vi "Locked Rotor.vi"(0 "GEA2 Reference In":refnum<k24>, 1 "Mode":T1, 2 "Hall Speed (RPM)":dbl=15.0, 3 "Previous Fault Count":u8, 5 "Standalone?":bool, 7 "GEA Inputs":T2={"Source"=228, "Destination"=32} {"Destination" format="%.0x"; "Source" format="%.0x"}, 11 "Error In":errorcluster, 12 "Counter":tag, 13 "Hall Sensor Channel":tag) -> (4 "GEA2 Reference Out":refnum<k24>, 6 "Pass/Fail?":bool, 8 "Report Text":string, 10 "Current Fault Count":u8, 15 "Error Out":errorcluster)   [LabVIEW 2016, in "TLMB.lvlib"]
doc: "This VI tests the locked rotor fault detection algorithm. It can be used to test in spin or agitate. QA XML must be used and test can only be executed on the soft load box (SLB)."
uses:
  Projects/TLMB.lvlib
  Q:/Common/DLLs/GEA3/GeaCommunication.dll
  Common/DLLs/GEA3/GeaCommunication.dll
  Common/LabVIEW GEA2 Toolkit/LabVIEW_GEA2_Toolkit.lvlibp/type defs/Source_Destination.ctl
  controls/Mode.ctl
  Common/LabVIEW GEA2 Toolkit/LabVIEW_GEA2_Toolkit.lvlibp/type defs/ERD Read Data In.ctl
  Common/LabVIEW GEA2 Toolkit/LabVIEW_GEA2_Toolkit.lvlibp/type defs/Data Type.ctl
  Common/LabVIEW GEA2 Toolkit/LabVIEW_GEA2_Toolkit.lvlibp/type defs/ERD Write Data In.ctl
  <vilib>/DAQmx/create/channels.llb/DAQmx Create Channel (CO-Pulse Generation-Frequency).vi
  <vilib>/DAQmx/configure/timing.llb/DAQmx Timing (Implicit).vi
  Common/LabVIEW GEA2 Toolkit/LabVIEW_GEA2_Toolkit.lvlibp
  <resource>/objmgr/daqmx.rc
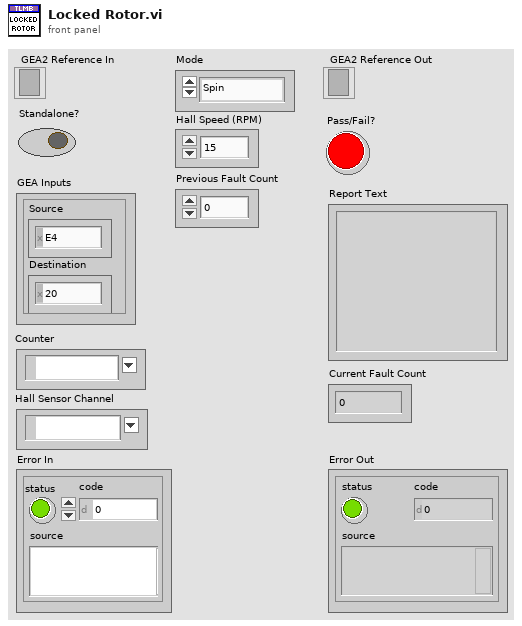
[diagram p1: front panel]
types:
  T1 = typedef "TLMB.lvlib/Mode.ctl" = enum16{"Spin", "Agitate"}
  T2 = typedef "LabVIEW_GEA2_Toolkit.lvlibp/Source_Destination.ctl" = cluster{"Source":u8, "Destination":u8}
  T3 = typedef "LabVIEW_GEA2_Toolkit.lvlibp/ERD Read Data In.ctl" = cluster{"ERD Number":u16, "Data Type":T4}
  T4 = typedef "LabVIEW_GEA2_Toolkit.lvlibp/Data Type.ctl" = enum16{"string", "boolean", "uint8_t", "uint16_t", "uint32_t", "uint64_t", "int8_t", "int16_t", "int32_t", "int64_t"}
  T5 = typedef "LabVIEW_GEA2_Toolkit.lvlibp/ERD Write Data In.ctl" = cluster{"ERD Number":u16, "Data Type":T4, "Data":string}
  T6 = typedef "LabVIEW_GEA2_Toolkit.lvlibp/ERD Read Data Out.ctl" = cluster{"ERD Number":u16, "Data":string}
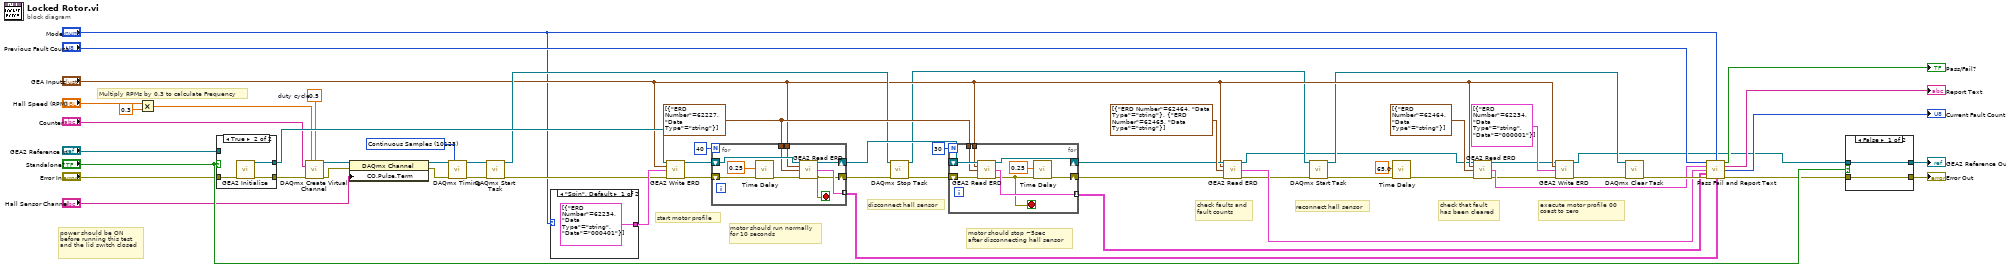
[diagram p0: block diagram]
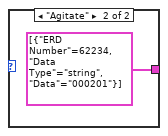
[diagram p2: hidden frame]
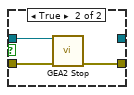
[diagram p3: hidden frame]
diagram:
  w42 = 0.5  # duty cycle
  w39 = T3[] [{"ERD Number"=62227, "Data Type"=enum."string"}] ("Read ERD List")
  w51 = 10123 items=["Finite Samples"=10178, "Continuous Samples"=10123, "Hardware Timed Single Point"=12522] ("sample mode")
  # "Multiply RPMs by 0.3 to calculate Frequency"
  # "check that fault\nhas been cleared"
  # "check faults and\nfault counts"
  # "reconnect hall sensor"
  # "power should be ON\nbefore running this test\nand the lid switch closed"
  # "execute motor profile 00\ncoast to zero"
  # "motor should stop ~5sec\nafter disconnecting hall sensor"
  # "start motor profile"
  # "motor should run normally\nfor 10 seconds"
  # "disconnect hall sensor"
  n1 = Multiply(x="Hall Speed (RPM)", y=0.3) -> (x*y=w43:dbl)
  n2 = case shown="True" "Standalone?" {
    tunnel: [w60 w64] -> w57
    tunnel: [w61 w63] -> w11
    tunnel: "Error In" -> [w61 w62]
    tunnel: "GEA2 Reference In" -> [w60 _]
    frame False {
    }
    frame True {
      n3 = call "GEA2 Initialize.vi"("error in"=w62) -> ("GEA2 Reference Out"=w64:refnum<k24>, "error out"=w63:errorcluster)  [unwired: 12 in, 1 out]
    }
  }
  n4 = call-poly <vilib>:"DAQmx Create Virtual Channel.vi"("frequency"=w43, "duty cycle"=w42, "counter"="Counter", "error in"=w11) -> ("task out"=w55:refnum<k21>, "error out"=w54:errorcluster)  [unwired: 10 in]
  n5 = property class="DAQmx Channel"(reference=w55, error in=w54, "CO.Pulse.Term"="Hall Sensor Channel") -> (reference out=w53:refnum<k21>, error out=w52:errorcluster)
  n6 = call-poly <vilib>:"DAQmx Timing.vi"("task/channels in"=w53, "sample mode"=w51, "error in"=w52) -> ("task out"=w50:refnum<k21>, "error out"=w49:errorcluster)  [unwired: 11 in]
  n7 = call <vilib>:"DAQmx Start Task.vi"("task/channels in"=w50, "error in"=w49) -> ("task out"=w33:refnum<k21>, "error out"=w48:errorcluster)  [unwired: 12 in]
  n8 = case shown="\"Spin\", Default" "Mode" {
    tunnel: [T5[] [{"ERD Number"=62234, "Data Type"=enum."string", "Data"="000401"}] ("Write ERD List") T5[] [{"ERD Number"=62234, "Data Type"=enum."string", "Data"="000201"}] ("Write ERD List")] -> w56
    frame "Spin", Default {
    }
    frame "Agitate" {
    }
  }
  n9 = call "GEA2 Write ERD.vi"("GEA2 Reference In"=w57, "GEA Inputs"="GEA Inputs", "Write ERD List"=w56, "Error In"=w48) -> ("GEA2 Reference Out"=w46:refnum<k24>, "Error Out"=w47:errorcluster)  [unwired: 9 in, 1 out]
  n10 = for {
    N: 40 -> [_]
    shift-right: [w67] -> w34
    shift-left: w47 -> [w70]
    shift-right: [w74] -> w40
    shift-left: w46 -> [w75]
    tunnel: "GEA Inputs" -> [w73]
    tunnel: w39 -> [w72]
    tunnel: [w68] -> w21 mode=indexing
    stop <- w67 stop-if-true
    n11 = call "Time Delay"("error in (no error)"=w70, "Delay Time (s)"=0.25) -> ("error out"=w69:errorcluster)  [unwired: 9 in]
    n12 = call "GEA2 Read ERD.vi"("GEA2 Reference In"=w75, "GEA Inputs"=w73, "Read ERD List"=w72, "Error In"=w69) -> ("GEA2 Reference Out"=w74:refnum<k24>, "ERD Data Out"=w68:T6[], "Error Out"=w67:errorcluster)  [unwired: 8 in, 1 out]
  }
  n13 = call <vilib>:"DAQmx Stop Task.vi"("task/channels in"=w33, "error in"=w34) -> ("task out"=w25:refnum<k21>, "error out"=w23:errorcluster)  [unwired: 12 in]
  n14 = for {
    N: 30 -> [_]
    shift-right: [w79] -> w37
    shift-left: w23 -> [w84]
    shift-right: [w82] -> w35
    shift-left: w40 -> [w83]
    tunnel: "GEA Inputs" -> [w81]
    tunnel: w39 -> [w80]
    tunnel: [w77] -> w20 mode=indexing
    stop <- w76 stop-if-true
    n15 = call "GEA2 Read ERD.vi"("GEA2 Reference In"=w83, "GEA Inputs"=w81, "Read ERD List"=w80, "Error In"=w84) -> ("GEA2 Reference Out"=w82:refnum<k24>, "ERD Data Out"=w77:T6[], "Error Out"=w76:errorcluster)  [unwired: 8 in, 1 out]
    n16 = call "Time Delay"("error in (no error)"=w76, "Delay Time (s)"=0.25) -> ("error out"=w79:errorcluster)  [unwired: 9 in]
  }
  n17 = call "GEA2 Read ERD.vi"("GEA2 Reference In"=w35, "GEA Inputs"="GEA Inputs", "Read ERD List"=T3[] [{"ERD Number"=62464, "Data Type"=enum."string"}, {"ERD Number"=62465, "Data Type"=enum."string"}], "Error In"=w37) -> ("GEA2 Reference Out"=w6:refnum<k24>, "ERD Data Out"=w19:T6[], "Error Out"=w7:errorcluster)  [unwired: 8 in, 1 out]
  n18 = call <vilib>:"DAQmx Start Task.vi"("task/channels in"=w25, "error in"=w7) -> ("task out"=w24:refnum<k21>, "error out"=w26:errorcluster)  [unwired: 12 in]
  n19 = call "Time Delay"("error in (no error)"=w26, "Delay Time (s)"=65.0) -> ("error out"=w29:errorcluster)  [unwired: 9 in]
  n20 = call "GEA2 Read ERD.vi"("GEA2 Reference In"=w6, "GEA Inputs"="GEA Inputs", "Read ERD List"=T3[] [{"ERD Number"=62464, "Data Type"=enum."string"}], "Error In"=w29) -> ("GEA2 Reference Out"=w10:refnum<k24>, "ERD Data Out"=w18:T6[], "Error Out"=w9:errorcluster)  [unwired: 8 in, 1 out]
  n21 = call "GEA2 Write ERD.vi"("GEA2 Reference In"=w10, "GEA Inputs"="GEA Inputs", "Write ERD List"=T5[] [{"ERD Number"=62234, "Data Type"=enum."string", "Data"="000001"}], "Error In"=w9) -> ("GEA2 Reference Out"=w5:refnum<k24>, "Error Out"=w8:errorcluster)  [unwired: 9 in, 1 out]
  n22 = call <vilib>:"DAQmx Clear Task.vi"("task in"=w24, "error in"=w8) -> ("error out"=w22:errorcluster)  [unwired: 13 in]
  n23 = call "Pass Fail and Report Text.vi"("Previous Fault Count"="Previous Fault Count", "Mode"="Mode", "Faults Cleared"=w18, "Faults Active"=w19, "Motor Stopped"=w20, "Error In"=w22, "Motor Running"=w21) -> ("Pass/Fail?"=→"Pass/Fail?":bool, "Report Text"=→"Report Text":string, "Current Fault Count"=→"Current Fault Count":u8, "Error Out"=w3:errorcluster)  [unwired: 5 in]
  n24 = case shown="False" "Standalone?" {
    tunnel: w3 -> [w86 w89]
    tunnel: [w86 w88] -> w27
    tunnel: w5 -> [w85 w87]
    tunnel: [w85 _] -> w14
    frame False {
    }
    frame True {
      n25 = call "GEA2 Stop.vi"("GEA2 Reference In"=w87, "Error In"=w89) -> ("Error Out"=w88:errorcluster)  [unwired: 13 in]
    }
  }
  "Error Out" <- w27
  "GEA2 Reference Out" <- w14
